vi "Accelerator DML Not Complex Process.vi"(9 "Sessions Parameters":T1={"intra_op_num_threads"=0, "inter_op_num_threads"=0, "execution_mode"=enum."ORT_SEQUENTIAL", "deterministic_compute"=FALSE, "graph_optimization_level"=1, "optimized_model_file_path"=path "", "profiling output dir"=path ""} {"graph_optimization_level" items=["ORT_DISABLE_ALL"=0, "ORT_ENABLE_ALL"=1, "ORT_ENABLE_BASIC"=2, "ORT_ENABLE_EXTENDED"=99]}, 11 "X size":i32=16384) -> (3 "Accelerator Time":dbl=0.19947869999998602)   [LabVIEW 2020]
uses:
  <vilib>/Graiphic/Accelerator/Source/Model/_Methods/acc_create_onnx_model_then_init_dml_inference_session.vi
  <vilib>/Graiphic/Accelerator/Source/SubVIs/add_to_cluster_onnx_input/acc_onnx_add_1d_float_array_into_input_cluster_array_by_idx.vi
  <vilib>/Graiphic/Accelerator/Source/SubVIs/add_to_cluster_onnx_input/acc_onnx_add_scalar_float_into_input_cluster_array_by_idx.vi
  <vilib>/Graiphic/Accelerator/Source/ONNX/Inference/_Methods/Simplified/acc_embedded_run_preallocated_multi_input_and_outputs_dml_by_idx.vi
  <vilib>/Graiphic/Accelerator/Source/ONNX/Inference/_Methods/Exec_DML/acc_embedded_copy_dml_ptr_data_to_labview_data.vi
  <vilib>/Graiphic/Accelerator/Source/ONNX/Inference/_Methods/Simplified/acc_embedded_run_mono_output_scalar_float.vi
  <vilib>/Graiphic/Accelerator/Source/ONNX/Inference/acc_Inference.lvclass
  <vilib>/Analysis/NI_AALBase.lvlib
  <vilib>/Graiphic/Accelerator/Source/Model/acc_Model.lvclass
panel:
  out "max value":sgl=5.4420166
  in  "nb_loop":i32=6
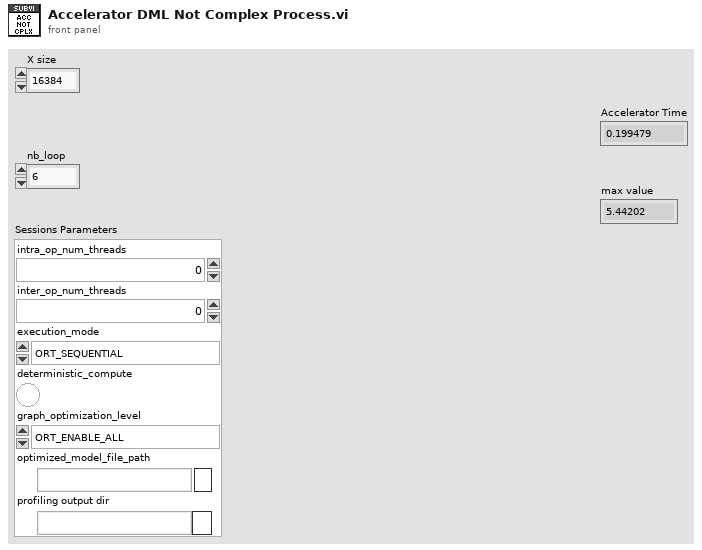
[diagram p1: front panel]
types:
  T1 = cluster{"intra_op_num_threads":i32, "inter_op_num_threads":i32, "execution_mode":enum16{"ORT_SEQUENTIAL", "ORT_PARALLEL"}, "deterministic_compute":bool, "graph_optimization_level":u16, "optimized_model_file_path":path, "profiling output dir":path}
  T2 = typedef "acc_onnx_multi_input_index_cluster.ctl" = cluster{"input_order":u32, "Inputs Info":cluster{"inputs_data":u8[], "inputs_shapes":i64[], "inputs string length":i64[], "inputs_ranks":i64[], "inputs_types":T3[]}}
  T3 = typedef "acc_onnx_dtype_enum.ctl" = enum16{"UNDEFINED", "FLOAT", "UINT8", "INT8", "UINT16", "INT16", "INT32", "INT64", "STRING", "BOOL", "FLOAT16", "DOUBLE", "UINT32", "UINT64", "COMPLEX64", "COMPLEX128", "BFLOAT16", "FLOAT8E4M3FN", "FLOAT8E4M3FNUZ", "FLOAT8E5M2", "FLOAT8E5M2FNUZ", "UINT4", "INT4"}
  T4 = typedef "acc_onnx_multi_ptr_input_index_cluster.ctl" = cluster{"input_order":u32, "Inputs Info":cluster{"inputs_ptr":u64, "inputs_shapes":i64[], "inputs_ranks":i64, "inputs_types":T3}}
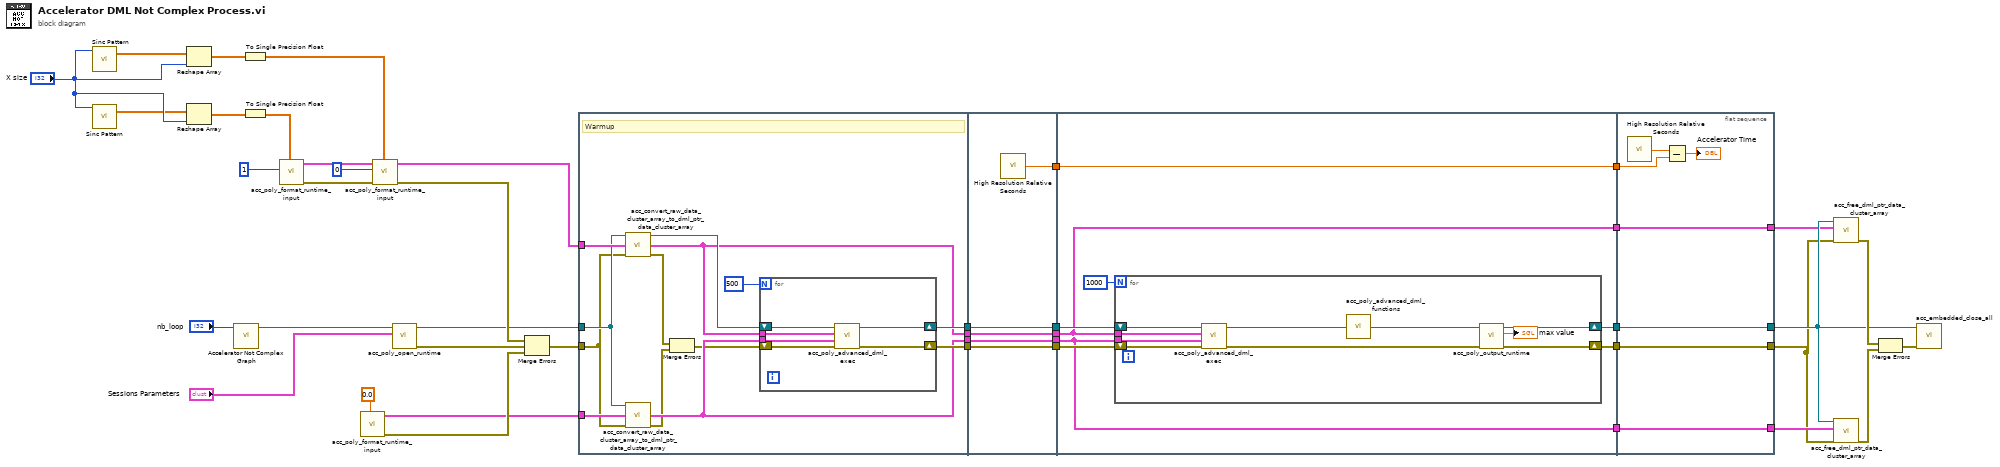
[diagram p0: block diagram]
diagram:
  n1 = call <vilib>:"Sinc Pattern.vi"("samples"="X size") -> ("Sinc Pattern"=w40:dbl[])  [unwired: 3 in, 1 out]
  n2 = call <vilib>:"Sinc Pattern.vi"("samples"="X size") -> ("Sinc Pattern"=w41:dbl[])  [unwired: 3 in, 1 out]
  n3 = Reshape Array(w40, "X size") -> (w2:dbl[])
  n4 = Reshape Array(w41, "X size") -> (w3:dbl[])
  n5 = call "Accelerator Not Complex Graph.vi"("nb_loop"="nb_loop") -> ("Model out"=w4:refnum<class "acc_Model.lvclass">)  [unwired: 10 in]
  n6 = To Single Precision Float(number=w2) -> (single precision float=w18:sgl[])
  n7 = To Single Precision Float(number=w3) -> (single precision float=w19:sgl[])
  n8 = call-poly <vilib>:"acc_poly_format_runtime_input.vi"("1D Input Data"=w19, "input order"=1) -> ("error out"=w22:errorcluster, "Data out (Fwd in)"=w23:T2[])  [unwired: 8 in]
  n9 = call-poly <vilib>:"acc_poly_format_runtime_input.vi"("Input Data"=sgl 0.0) -> ("error out"=w20:errorcluster, "Data out (Fwd in)"=w12:T2[])  [unwired: 9 in]
  n10 = call-poly <vilib>:"acc_poly_format_runtime_input.vi"("1D Input Data"=w18, "error in"=w22, "input order"=0, "Data in"=w23) -> ("error out"=w21:errorcluster, "Data out (Fwd in)"=w15:T2[])  [unwired: 6 in]
  n11 = call-poly <vilib>:"acc_poly_open_runtime.vi"("Sessions Parameters"="Sessions Parameters", "Model in"=w4) -> ("error out"=w17:errorcluster, "Inference out"=w13:refnum<class "acc_Inference.lvclass">)  [unwired: 8 in]
  n12 = Merge Errors(w21, w17, w20) -> (w14:errorcluster)
  n13 = flat-sequence {
    tunnel: w14 -> [w47]
    tunnel: w15 -> [w52]
    tunnel: w12 -> [w51]
    tunnel: w13 -> [w50]
    tunnel: [w56] -> w39
    tunnel: [w49] -> w38
    tunnel: [w55] -> w37
    tunnel: [w48] -> w36
    tunnel: [w67] -> w35
    tunnel: [w66] -> w34
    tunnel: [w65] -> w33
    tunnel: [w64] -> w32
    tunnel: [w63] -> w31
    tunnel: w39 -> [w66]
    tunnel: w38 -> [w65]
    tunnel: w37 -> [w63]
    tunnel: w36 -> [w64]
    tunnel: w35 -> [w75]
    tunnel: [w75] -> w30
    tunnel: w34 -> [w73]
    tunnel: w33 -> [w68]
    tunnel: w32 -> [w69]
    tunnel: w31 -> [w72]
    tunnel: [w71] -> w29
    tunnel: [w70] -> w28
    tunnel: [w69] -> w27
    tunnel: [w68] -> w26
    tunnel: w30 -> [w91]
    tunnel: [w89] -> w7
    tunnel: w29 -> [w89]
    tunnel: w28 -> [w88]
    tunnel: [w88] -> w6
    tunnel: [w87] -> w5
    tunnel: w27 -> [w87]
    tunnel: [w86] -> w8
    tunnel: w26 -> [w86]
    frame #0 {
      # "Warmup"
      n14 = call <vilib>:"acc_convert_raw_data_cluster_array_to_dml_ptr_data_cluster_array.vi"("Inference in"=w50, "Data in"=w52, "error in"=w47) -> ("Inference out"=w53:refnum<class "acc_Inference.lvclass">, "Data in"=w48:T4[], "error out"=w44:errorcluster)  [unwired: 10 in]
      n15 = call <vilib>:"acc_convert_raw_data_cluster_array_to_dml_ptr_data_cluster_array.vi"("Inference in"=w50, "Data in"=w51, "error in"=w47) -> ("Data in"=w49:T4[], "error out"=w46:errorcluster)  [unwired: 10 in, 1 out]
      n16 = Merge Errors(w44, w46) -> (w45:errorcluster)
      n17 = for {
        N: 500 -> [_]
        tunnel: w48 -> [w59]
        tunnel: w49 -> [w58]
        shift-right: [w61] -> w56
        shift-left: w53 -> [w62]
        shift-right: [w57] -> w55
        shift-left: w45 -> [w60]
        n18 = call-poly <vilib>:"acc_poly_advanced_dml_exec.vi"("error in"=w60, "Data out"=w58, "Data in"=w59, "Inference in"=w62) -> ("error out"=w57:errorcluster, "Inference out"=w61:refnum<class "acc_Inference.lvclass">)  [unwired: 6 in]
      }
    }
    frame #1 {
      n19 = call <vilib>:"High Resolution Relative Seconds.vi"() -> ("relative seconds"=w67:dbl)
    }
    frame #2 {
      n20 = for {
        N: 1000 -> [_]
        tunnel: w68 -> [w84]
        tunnel: w69 -> [w83]
        shift-right: [w79] -> w71
        shift-left: w73 -> [w85]
        shift-right: [w78] -> w70
        shift-left: w72 -> [w82]
        n21 = call-poly <vilib>:"acc_poly_advanced_dml_exec.vi"("error in"=w82, "Data out"=w84, "Data in"=w83, "Inference in"=w85) -> ("error out"=w80:errorcluster, "Inference out"=w81:refnum<class "acc_Inference.lvclass">)  [unwired: 6 in]
        n22 = call-poly <vilib>:"acc_poly_advanced_dml_functions.vi"("Inference in"=w81) -> ("Inference out"=w77:refnum<class "acc_Inference.lvclass">)
        n23 = call-poly <vilib>:"acc_poly_output_runtime.vi"("error in"=w80, "Inference in"=w77) -> ("error out"=w78:errorcluster, "Output Data"=→"max value":sgl, "Inference out"=w79:refnum<class "acc_Inference.lvclass">)  [unwired: 7 in]
      }
    }
    frame #3 {
      n24 = call <vilib>:"High Resolution Relative Seconds.vi"() -> ("relative seconds"=w92:dbl)
      n25 = Subtract(x=w92, y=w91) -> (x-y=→"Accelerator Time":dbl)
    }
  }
  n26 = call <vilib>:"acc_free_dml_ptr_data_cluster_array.vi"("error in"=w6, "Data in"=w5, "Inference in"=w7) -> ("error out"=w10:errorcluster)  [unwired: 7 in, 1 out]
  n27 = call <vilib>:"acc_free_dml_ptr_data_cluster_array.vi"("error in"=w6, "Data in"=w8, "Inference in"=w7) -> ("error out"=w11:errorcluster)  [unwired: 7 in, 1 out]
  n28 = Merge Errors(w10, w11) -> (w9:errorcluster)
  n29 = call-dynamic "acc_embedded_close_all.vi"("error in"=w9, "Inference in"=w7) -> ()  [unwired: 8 in, 2 out]
